vi "Stop sweep.vi"(7 "Status":enum16{"Set", "Get", "Reset"}(ring), 8 "Error In":errorcluster, 10 "Exit?":bool) -> (0 "Error Out":errorcluster, 2 "Exit?":bool)   [LabVIEW 2016]
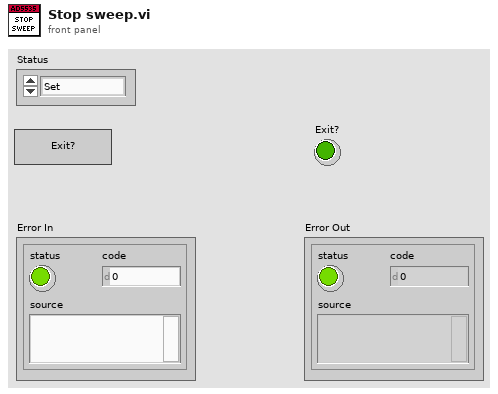
[diagram p1: front panel]
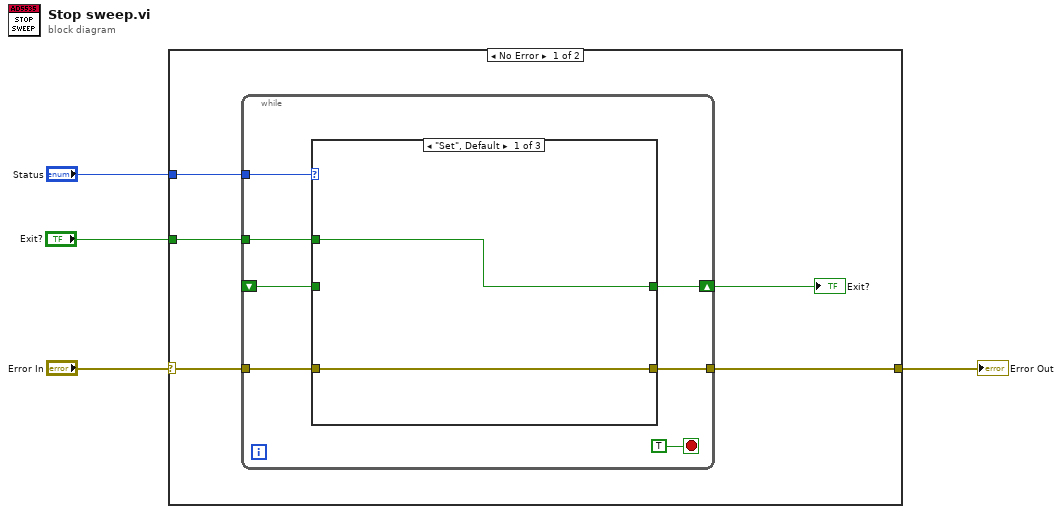
[diagram p0: block diagram]
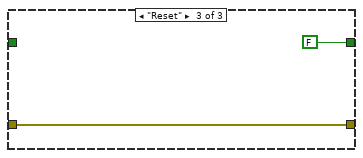
[diagram p3: hidden frame]
diagram:
  n1 = case shown="No Error" "Error In" {
    selector: "Error In" -> [w6 w23]
    tunnel: [w7 w23] -> w3
    tunnel: "Status" -> [w9 _]
    tunnel: "Exit?" -> [w8 _]
    frame No Error {
      n2 = while {
        tunnel: w9 -> [w15]
        shift-right: [w14] -> w5
        shift-left: _ -> [w12]
        tunnel: w8 -> [w13]
        tunnel: [w11] -> w7
        tunnel: w6 -> [w10]
        stop <- TRUE stop-if-true
        n3 = case shown="\"Set\", Default" w15 {
          tunnel: [w18 w19 FALSE ("Exit?")] -> w14
          tunnel: w13 -> [w18 _ _]
          tunnel: w12 -> [_ w19 _]
          tunnel: [w17 w20 w21] -> w11
          tunnel: w10 -> [w17 w20 w21]
          frame "Set", Default {
          }
          frame "Get" {
          }
          frame "Reset" {
          }
        }
      }
      "Exit?" <- w5
    }
    frame Error {
    }
  }
  "Error Out" <- w3
